vi "Set Format.vi"(8 "error in":errorcluster, 10 "Format":string="%s - %-7s - %s - %s - %d - %s\\n", 11 "Formatter in":refnum<class "Formatter.lvclass">) -> (0 "error out":errorcluster, 3 "Formatter out":refnum<class "Formatter.lvclass">)   [LabVIEW 2016, in "hse-logger.lvlib" / "Formatter.lvclass"]
doc: "A format string in the given style for the logged output as a whole. The possible mapping keys are drawn from the LogRecord object’s LogRecord attributes. If not specified, \"%s - %-7s - %s - %s - %d - %s\\n\" is used which corresponds to Time - Level - Callchain - Message - Error Code - Error Message."
uses:
  Formatter.lvclass
  Formatter.lvclass/Formatter.ctl
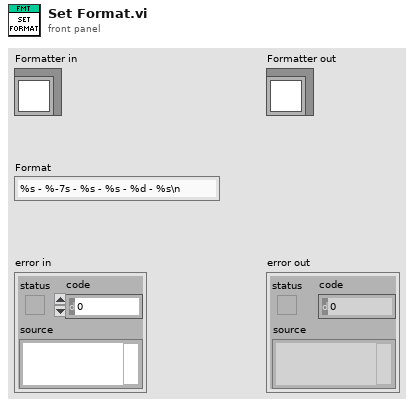
[diagram p1: front panel]
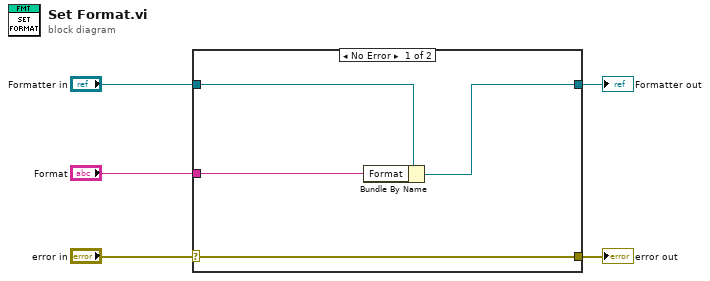
[diagram p0: block diagram]
diagram:
  n1 = case shown="No Error" "error in" {
    selector: "error in" -> [w9 w11]
    tunnel: [w9 w11] -> w4
    tunnel: [w7 w10] -> w2
    tunnel: "Formatter in" -> [w8 w10]
    tunnel: "Format" -> [w6 _]
    frame No Error {
      n2 = Bundle By Name(cluster=w8, "Format"=w6) -> (w7:refnum<class "Formatter.lvclass">)
    }
    frame Error {
    }
  }
  "error out" <- w4
  "Formatter out" <- w2
